vi "Cubic Spline Generator.vi"(1 "Configurations":cluster{"Xf":dbl, "Xo":dbl, "Vf":dbl, "Vo":dbl}) -> (0 "Spline":dbl[](array[numeric]))   [LabVIEW 2016]
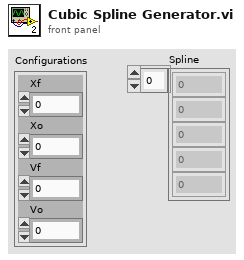
[diagram p1: front panel]
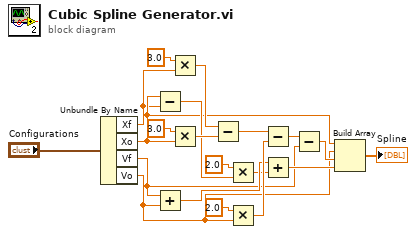
[diagram p0: block diagram]
diagram:
  n1 = Unbundle By Name("Configurations") -> ("Xf"=w1:dbl, "Xo"=w4:dbl, "Vf"=w3:dbl, "Vo"=w2:dbl)
  n2 = Subtract(x=w4, y=w1) -> (x-y=w11:dbl)
  n3 = Add(x=w3, y=w2) -> (x+y=w10:dbl)
  n4 = Multiply(x=3.0, y=w1) -> (x*y=w18:dbl)
  n5 = Multiply(x=3.0, y=w4) -> (x*y=w17:dbl)
  n6 = Subtract(x=w18, y=w17) -> (x-y=w15:dbl)
  n7 = Multiply(x=2.0, y=w11) -> (x*y=w9:dbl)
  n8 = Multiply(x=2.0, y=w2) -> (x*y=w14:dbl)
  n9 = Subtract(x=w15, y=w14) -> (x-y=w13:dbl)
  n10 = Add(x=w10, y=w9) -> (x+y=w7:dbl)
  n11 = Subtract(x=w13, y=w3) -> (x-y=w6:dbl)
  n12 = Build Array(w4, w2, w6, w7) -> (→"Spline":dbl[])
